vi "oneMotor.vi"() -> ()   [LabVIEW 2019]
panel:
  in  "stop":bool
  in  "DC_Pwr":dbl[](array[numeric])
  out "ENC":i32[](array[numeric])
  in  "Reset Counter":bool
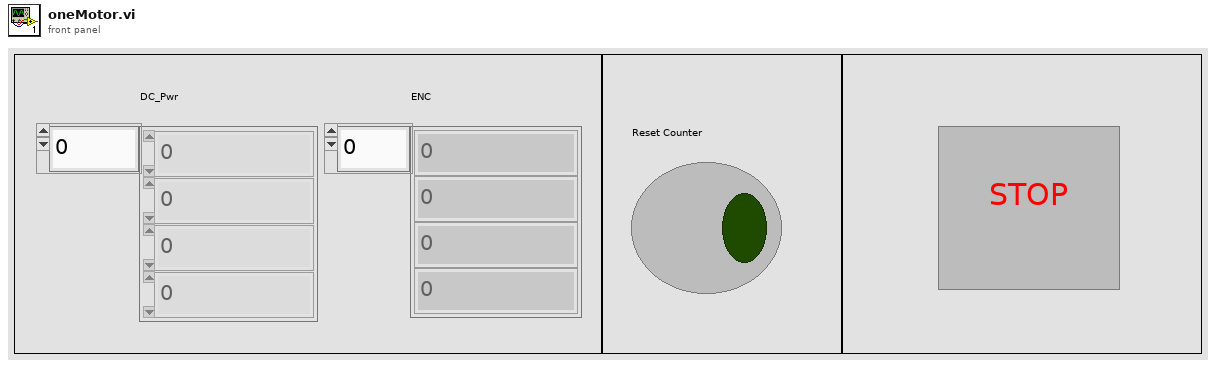
[diagram p1: front panel]
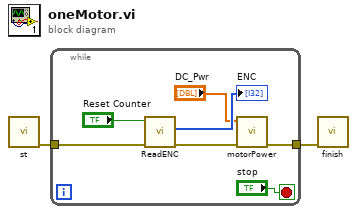
[diagram p0: block diagram]
diagram:
  n1 = call "st.vi"() -> ("Error/Flow Out"=w2:errorcluster)  [unwired: 11 in]
  n2 = while {
    tunnel: w2 -> [w8]
    tunnel: [w3] -> w1
    stop <- "stop" stop-if-true
    n3 = call "ReadENC.vi"("error in (no error)"=w8, "Reset"="Reset Counter") -> ("error out"=w4:errorcluster, "ENC"=→"ENC":i32[])  [unwired: 8 in]
    n4 = call "motorPower.vi"("error in (no error)"=w4, "DC_Pwr"="DC_Pwr") -> ("error out"=w3:errorcluster)  [unwired: 9 in]
  }
  n5 = call "finish.vi"("Error/Flow In"=w1) -> ()  [unwired: 11 in]
